vi "Cycle Selection_Run.vi"(0 "GEA2 Reference In":refnum<k24>, 5 "Option Selection":T2, 7 "ECT Parameters":T1={"MS to Spin Time"=0, "Target Fill Time"=0, "MS to Agitate Time"=0, "MS to Spin before Spin Time "=0, "Adaptive Drain Time"=60, "Coast to 0 Time"=60}, 11 "Error In":errorcluster) -> (4 "GEA2 Reference Out":refnum<k24>, 6 "Machine State Pass/Fail":bool, 8 "Report text":string, 15 "Error Out":errorcluster)   [LabVIEW 2016, in "TL27.lvlib"]
doc: "This vi can be used to read ERD every 1 sec for user selected repeat counts."
uses:
  Projects/TL27.lvlib
  C:/Automation/DLLs/PC Dot Net/GeaCommunication.dll
  Controls/Options.ctl
  Controls/ECT Parameters.ctl
  Common/LabVIEW GEA2 Toolkit/LabVIEW_GEA2_Toolkit.lvlibp/type defs/Source_Destination.ctl
  Valew Common/type defs/Encoder Position.ctl
  Common/LabVIEW GEA2 Toolkit/LabVIEW_GEA2_Toolkit.lvlibp/type defs/ERD Write Data In.ctl
  Common/LabVIEW GEA2 Toolkit/LabVIEW_GEA2_Toolkit.lvlibp/type defs/Data Type.ctl
  Valew Common/type defs/UI Buttons.ctl
  Common/LabVIEW GEA2 Toolkit/LabVIEW_GEA2_Toolkit.lvlibp/type defs/ERD Read Data In.ctl
  Common/LabVIEW GEA2 Toolkit/LabVIEW_GEA2_Toolkit.lvlibp
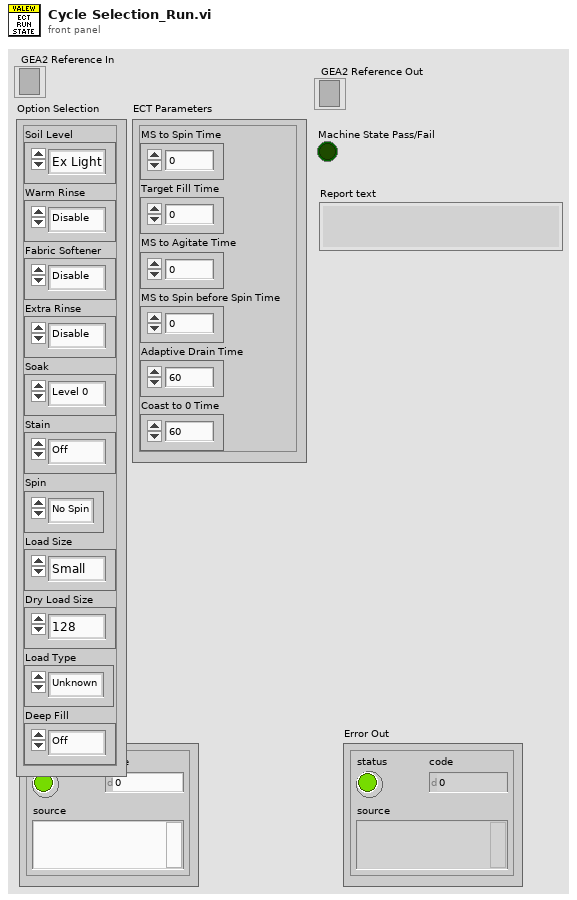
[diagram p1: front panel]
types:
  T1 = typedef "TL27.lvlib/ECT Parameters.ctl" = cluster{"MS to Spin Time":u16, "Target Fill Time":u16, "MS to Agitate Time":u16, "MS to Spin before Spin Time ":u16, "Adaptive Drain Time":u16, "Coast to 0 Time":u16}
  T2 = typedef "TL27.lvlib/Options.ctl" = cluster{"Soil Level":enum8{"Ex Light", "Light", "Normal", "Heavy", "Ex Heavy"}, "Warm Rinse":enum8{"Disable", "Enable"}, "Fabric Softener":enum16{"Disable", "Enable"}, "Extra Rinse":enum8{"Disable", "Enable"}, "Soak":enum8{"Level 0", "Level 1", "Level 2", "Level 3", "Level 4"}, "Stain":enum8{"Off", "Tomato", "Wine", "Blood", "Grass", "Dirt"}, "Spin":enum16{"No Spin", "Normal Spin", "More Spin", "Max Spin"}, "Load Size":enum8{"Small", "Medium", "Large", "Super", "Precise Fill", "Super Plus"}, "Dry Load Size":enum16{"128", "256", "384", "5AA", "6A4", "834", "65535"}, "Load Type":enum8{"Unknown", "Cotton", "Synthetic", "Mixed", "Wet", "Low Flow", "Small", "Medium", "Large", "Super", "Super Plus", "Max"}, "Deep Fill":enum8{"Off", "Incremental Fill", "Max Fill"}}
  T3 = typedef "LabVIEW_GEA2_Toolkit.lvlibp/Source_Destination.ctl" = cluster{"Source":u8, "Destination":u8}
  T4 = typedef "LabVIEW_GEA2_Toolkit.lvlibp/ERD Read Data In.ctl" = cluster{"ERD Number":u16, "Data Type":T5}
  T5 = typedef "LabVIEW_GEA2_Toolkit.lvlibp/Data Type.ctl" = enum16{"string", "boolean", "uint8_t", "uint16_t", "uint32_t", "uint64_t", "int8_t", "int16_t", "int32_t", "int64_t"}
  T6 = typedef "TL27.lvlib/UI Buttons.ctl" = enum16{"Switch Off", "SW201 - My Cycle", "SW202 - Delay Wash", "SW203 - Extra Rinse", "SW204 - Signal / Volume", "SW205 - Spin", "SW206 - Deep Rinse / Fab Soft", "SW207 - Soil", "SW208 - Auto Soak", "SW209 - Temp", "SW210 - Warm Rinse", "SW211 - Deep Fill", "SW212 - Stain Remover", "SW213 - Power", "SW222 - Control Lock", "SW214 - Start / Pause", "SW301 - Start/Pause LE", "SW302 - Option Button LE", "SW201/212 - Bulk Flush"}
  T7 = typedef "LabVIEW_GEA2_Toolkit.lvlibp/ERD Write Data In.ctl" = cluster{"ERD Number":u16, "Data Type":T5, "Data":string}
  T8 = typedef "TL27.lvlib/Encoder Position.ctl" = enum16{"Position 0", "Position 1", "Position 2", "Position 3", "Position 4", "Position 5", "Position 6", "Position 7", "Position 8", "Position 9", "Position 10", "Position 11", "Position 12", "Position 13", "Clear / Reset"}
  T9 = typedef "TL27.lvlib/ECT.ctl" = cluster{"MS to Agitate Time":u16, "Adaptive Drain Time":u16, "Coast to 0 Time":u16, "Agitate Time":u16, "Warm Rinse Time":u16, "FS Time":u16, "Ex Rinse Time":u16, "Soak Time":u16, "Stain Time":u16, "Motor Profile ID":u16, "Calculated ECT":u16, "Spin Time":u16}
  T10 = typedef "LabVIEW_GEA2_Toolkit.lvlibp/ERD Read Data Out.ctl" = cluster{"ERD Number":u16, "Data":string}
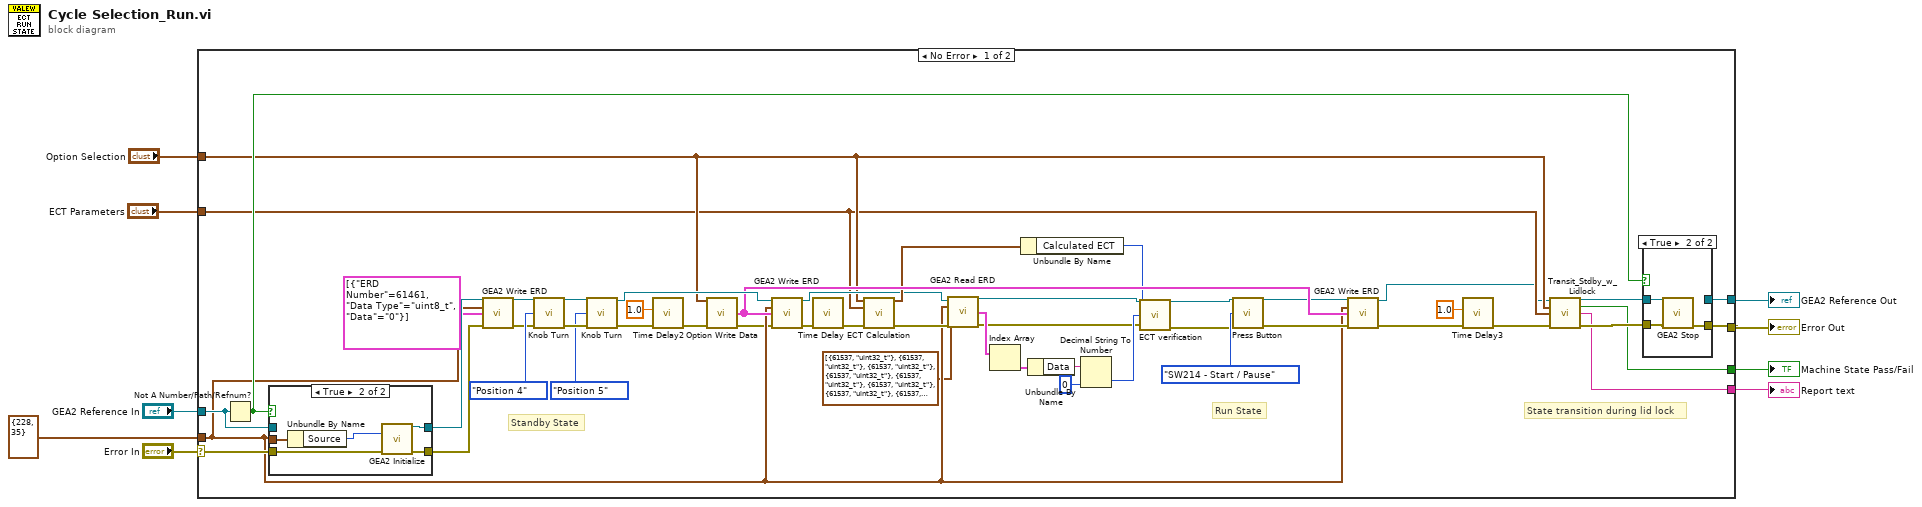
[diagram p0: block diagram]
diagram:
  n1 = case shown="No Error" "Error In" {
    selector: "Error In" -> [w58 w72]
    tunnel: T3 {"Source"=228, "Destination"=35} ("GEA Inputs") -> [w25 _]
    tunnel: "GEA2 Reference In" -> [w59 w73]
    tunnel: [w26 w73] -> w6
    tunnel: [w40 w72] -> w5
    tunnel: "Option Selection" -> [w20 _]
    tunnel: [w24 _] -> w3
    tunnel: [w23 _] -> w2
    tunnel: "ECT Parameters" -> [w15 _]
    frame No Error {
      # "State transition during lid lock"
      # "Run State"
      # "Standby State"
      n2 = Not A Number/Path/Refnum?(number/path/refnum=w59) -> (NaN/Path/Refnum?=w47:bool)
      n3 = case shown="True" w47 {
        tunnel: w58 -> [w66 w71]
        tunnel: [w66 w70] -> w53
        tunnel: [w65 w69] -> w52
        tunnel: w25 -> [_ w67]
        tunnel: w59 -> [w65 _]
        frame False {
        }
        frame True {
          n4 = Unbundle By Name(w67) -> ("Source"=w68:u8)
          n5 = call "GEA2 Initialize.vi"("Source Address"=w68, "error in"=w71) -> ("GEA2 Reference Out"=w69:refnum<k24>, "error out"=w70:errorcluster)  [unwired: 11 in, 1 out]
        }
      }
      n6 = call "GEA2 Write ERD.vi"("GEA2 Reference In"=w52, "GEA Inputs"=w25, "Write ERD List"=T7[] [{"ERD Number"=61461, "Data Type"=enum."uint8_t", "Data"="0"}], "Error In"=w53) -> ("GEA2 Reference Out"=w51:refnum<k24>, "Error Out"=w50:errorcluster)  [unwired: 9 in, 1 out]
      n7 = call "Knob Turn.vi"("GEA2 Reference In"=w51, "Button"=Encoder_Position."Position 4", "Error In"=w50) -> ("GEA2 Reference Out"=w56:refnum<k24>, "Error Out"=w55:errorcluster)  [unwired: 11 in]
      n8 = call "Knob Turn.vi"("GEA2 Reference In"=w56, "Button"=Encoder_Position."Position 5", "Error In"=w55) -> ("GEA2 Reference Out"=w46:refnum<k24>, "Error Out"=w19:errorcluster)  [unwired: 11 in]
      n9 = call "Time Delay2"("error in (no error)"=w19, "Delay Time (s)"=1.0) -> ("error out"=w17:errorcluster)  [unwired: 9 in]
      n10 = call "Option Write Data.vi"("Option Selection"=w20, "Error In"=w17) -> ("appended array"=w44:T7[], "Error Out"=w16:errorcluster)  [unwired: 12 in]
      n11 = call "GEA2 Write ERD.vi"("GEA2 Reference In"=w46, "GEA Inputs"=w25, "Write ERD List"=w44, "Error In"=w16) -> ("GEA2 Reference Out"=w21:refnum<k24>, "Error Out"=w48:errorcluster)  [unwired: 9 in, 1 out]
      n12 = call "Time Delay"("error in (no error)"=w48) -> ("error out"=w37:errorcluster)  [unwired: 10 in]
      n13 = call "ECT Calculation.vi"("Option Selection"=w20, "ECT Parameters"=w15, "Error In"=w37) -> ("Expected ECT"=w22:T9, "Error Out"=w30:errorcluster)  [unwired: 11 in]
      n14 = call "GEA2 Read ERD.vi"("GEA2 Reference In"=w21, "GEA Inputs"=w25, "Read ERD List"=T4[] [{"ERD Number"=61537, "Data Type"=enum."uint32_t"}, {"ERD Number"=61537, "Data Type"=enum."uint32_t"}, {"ERD Number"=61537, "Data Type"=enum."uint32_t"}, {"ERD Number"=61537, "Data Type"=enum."uint32_t"}, {"ERD Number"=61537, "Data Type"=enum."uint32_t"}, {"ERD Number"=61537, "Data Type"=enum."uint32_t"}, {"ERD Number"=61537, "Data Type"=enum."uint32_t"}, {"ERD Number"=61537, "Data Type"=enum."uint32_t"}], "Error In"=w30) -> ("GEA2 Reference Out"=w31:refnum<k24>, "ERD Data Out"=w36:T10[], "Error Out"=w29:errorcluster)  [unwired: 8 in, 1 out]
      n15 = Index Array(array=w36) -> (element=w35:T10)  [unwired: 1 in]
      n16 = Unbundle By Name(w22) -> ("Calculated ECT"=w32:u16)
      n17 = Unbundle By Name(w35) -> ("Data"=w34:string)
      n18 = Decimal String To Number(string=w34, default (0L)=u16 0 ("default (0 I32)")) -> (number=w33:u16)  [unwired: 1 in, 1 out]
      n19 = call "ECT verification.vi"(".NET Refnum in"=w31, "Cal ECT (sec)"=w32, "Time remaining (sec)"=w33, "error in"=w29) -> (".NET Refnum out"=w39:refnum<k24>, "error out"=w38:errorcluster)  [unwired: 5 in, 5 out]
      n20 = call "Press Button.vi"("GEA2 Reference In"=w39, "Button"=UI_Buttons."SW214 - Start / Pause", "Error In"=w38) -> ("GEA2 Reference Out"=w43:refnum<k24>, "Error Out"=w42:errorcluster)  [unwired: 11 in]
      n21 = call "GEA2 Write ERD.vi"("GEA2 Reference In"=w43, "GEA Inputs"=w25, "Write ERD List"=w44, "Error In"=w42) -> ("GEA2 Reference Out"=w12:refnum<k24>, "Error Out"=w41:errorcluster)  [unwired: 9 in, 1 out]
      n22 = call "Time Delay3"("error in (no error)"=w41, "Delay Time (s)"=1.0) -> ("error out"=w13:errorcluster)  [unwired: 9 in]
      n23 = call "Transit_Stdby_w_Lidlock.vi"("GEA2 Reference In"=w12, "Option Selection"=w20, "ECT Parameters"=w15, "Error In"=w13) -> ("GEA2 Reference Out"=w28:refnum<k24>, "Machine State Pass/Fail"=w24:bool, "Report text"=w23:string, "Error Out"=w27:errorcluster)  [unwired: 8 in]
      n24 = case shown="True" w47 {
        tunnel: [w60 w64] -> w40
        tunnel: w28 -> [w61 w63]
        tunnel: w27 -> [w60 w62]
        tunnel: [w61 _] -> w26
        frame False {
        }
        frame True {
          n25 = call "GEA2 Stop.vi"("GEA2 Reference In"=w63, "Error In"=w62) -> ("Error Out"=w64:errorcluster)  [unwired: 13 in]
        }
      }
    }
    frame Error {
    }
  }
  "GEA2 Reference Out" <- w6
  "Error Out" <- w5
  "Machine State Pass/Fail" <- w3
  "Report text" <- w2
